vi "Show Packages Folder.vi"(8 "Error In":errorcluster, 11 "Target Project Root":path) -> (0 "Error Out":errorcluster)   [LabVIEW 2017]
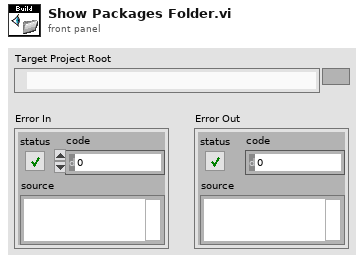
[diagram p1: front panel]
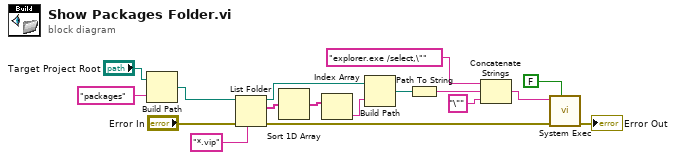
[diagram p0: block diagram]
diagram:
  n1 = Build Path(base path="Target Project Root", name or relative path="packages") -> (appended path=w9:path)
  n2 = List Folder(path=w9, pattern="*.vip", error in="Error In") -> (path out=w4:path, filenames=w2:string[], error out=w7:errorcluster)  [unwired: 1 in, 1 out]
  n3 = Sort 1D Array(array=w2) -> (sorted array=w1:string[])
  n4 = Index Array(array=w1) -> (element=w5:string)  [unwired: 1 in]
  n5 = Build Path(base path=w4, name or relative path=w5) -> (appended path=w3:path)
  n6 = Path To String(path=w3) -> (string=w14:string)
  n7 = Concatenate Strings("explorer.exe /select,\"" ("string"), w14, "\"" ("string")) -> (w12:string)
  n8 = call <vilib>:"System Exec.vi"("wait until completion? (T)"=FALSE, "error in (no error)"=w7, "command line"=w12) -> ("error out"=→"Error Out":errorcluster)  [unwired: 5 in, 3 out]
